vi "MainTestDemo.vi"() -> ()   [LabVIEW 2012]
uses:
  <userlib>/ROSforLV/ROS/Code/SubVIs/_ROSDirection.ctl
  <userlib>/ROSforLV/ROS/Code/_ROSDefinition.vi
  <userlib>/ROSforLV/ROS/parsing/std_msgs/subs/parse_time_scalar.vi
panel:
  in  "Tab Control":T1(tab)
  out "Time":cluster{"secs":i32, "nsecs":i32}
  in  "Load Boxes":bool
  out "WorldProperties":T2
  out "link names":string[](array[string])
  out "Link Poses":T3(array[cluster]) {"Point"."y" format="%#_3f"}
  out "Link Twists":T4(array[cluster])
  out "link names 2":string[](array[string])
  out "Link Twists 2":T4(array[cluster])
  out "Link Poses 2":T3(array[cluster]) {"Point"."y" format="%#_3f"}
  in  "Twist 2":T5
  in  "Pose 2":T6 {"Point"."x" scale=-3.0..3.0}
  in  "Pose":T6 {"Point"."x" scale=-3.0..3.0}
  in  "Twist":T5
  in  "Boolean":bool
  in  "stop":bool
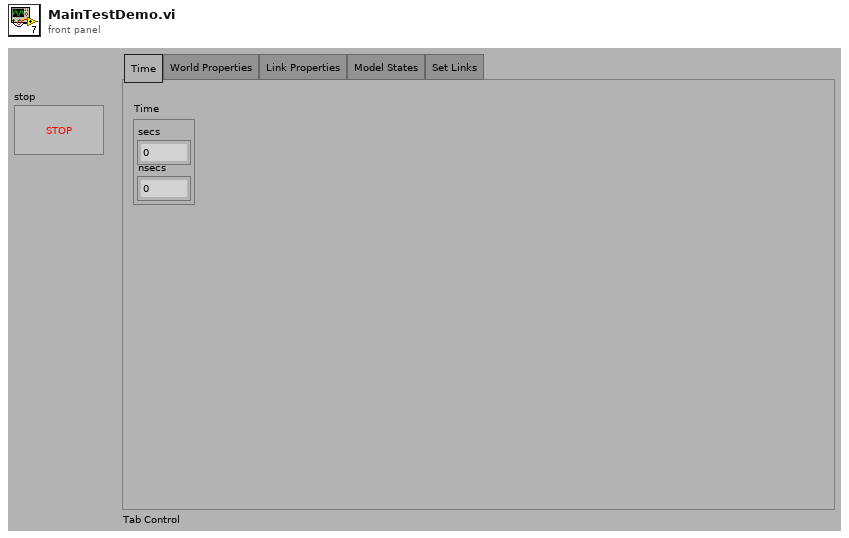
[diagram p1: front panel]
types:
  T1 = enum32{"Time", "World Properties", "Link Properties", "Model States", "Set Links"}
  T2 = cluster{"sim_time":dbl, "model_names":string[], "rendering enabled":bool, "success":bool, "status message":string}
  T3 = cluster{"Point":cluster{"x":dbl, "y":dbl, "z":dbl}, "Quaternion":cluster{"x":dbl, "y":dbl, "z":dbl, "w":dbl}}[]
  T4 = cluster{"Linear":cluster{"x":dbl, "y":dbl, "z":dbl}, "Angular":cluster{"x":dbl, "y":dbl, "z":dbl}}[]
  T5 = cluster{"Linear":cluster{"x":dbl, "y":dbl, "z":dbl}, "Angular":cluster{"x":dbl, "y":dbl, "z":dbl}}
  T6 = cluster{"Point":cluster{"x":dbl, "y":dbl, "z":dbl}, "Quaternion":cluster{"x":dbl, "y":dbl, "z":dbl, "w":dbl}}
  T7 = typedef "_ROSDirection.ctl" = enum16{"Node", "Publisher", "Subscriber", "Service Client"}
  T8 = cluster{"Topic":string, "Type":string, "Action":T7, "Update (ms)":u16, "write queue":u16}
  T9 = typedef "_ROSControl.ctl" = cluster{"topic port":u16, "Node":string, "topic":string, "type":string, "node port":u32, "error ":errorcluster, "Direction":T7, "APIs":string[], "Update (ms)":u16, "write queue":u16}
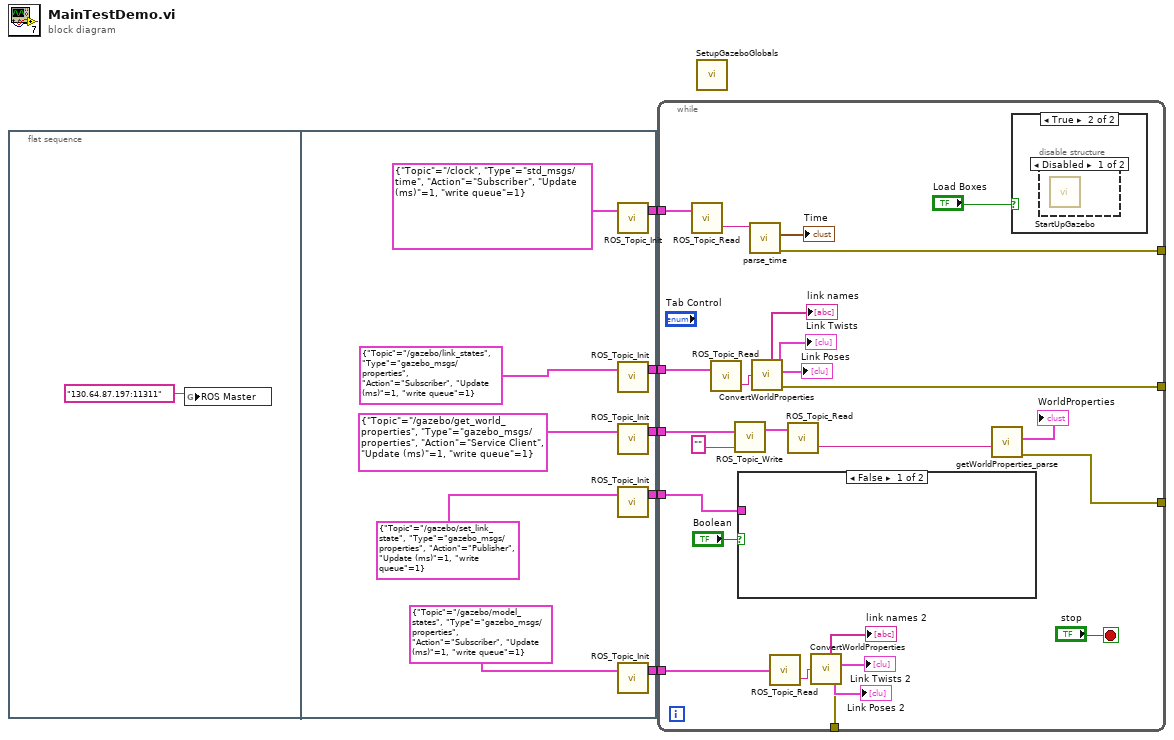
[diagram p0: block diagram]
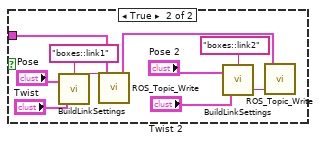
[diagram p2: hidden frame]
diagram:
  n1 = flat-sequence {
    tunnel: [w16] -> w5
    tunnel: [w15] -> w4
    tunnel: [w14] -> w3
    tunnel: [w13] -> w2
    tunnel: [w12] -> w1
    frame #0 {
      n2 = global write "_ROSDefinition.vi" "ROS Master"("130.64.87.197:11311" ("ROS Master")) -> ()
    }
    frame #1 {
      n3 = call <userlib>:"ROS_Topic_Init.vi"("Definitions"=T8 {"Topic"="/clock", "Type"="std_msgs/time", "Action"=enum."Subscriber", "Update (ms)"=1, "write queue"=1} ("element")) -> ("ROS out"=w16:T9)  [unwired: 2 in]
      n4 = call <userlib>:"ROS_Topic_Init.vi"("Definitions"=T8 {"Topic"="/gazebo/link_states", "Type"="gazebo_msgs/properties", "Action"=enum."Subscriber", "Update (ms)"=1, "write queue"=1} ("element")) -> ("ROS out"=w14:T9)  [unwired: 2 in]
      n5 = call <userlib>:"ROS_Topic_Init.vi"("Definitions"=T8 {"Topic"="/gazebo/get_world_properties", "Type"="gazebo_msgs/properties", "Action"=enum."Service Client", "Update (ms)"=1, "write queue"=1} ("element")) -> ("ROS out"=w15:T9)  [unwired: 2 in]
      n6 = call <userlib>:"ROS_Topic_Init.vi"("Definitions"=T8 {"Topic"="/gazebo/set_link_state", "Type"="gazebo_msgs/properties", "Action"=enum."Publisher", "Update (ms)"=1, "write queue"=1} ("element")) -> ("ROS out"=w13:T9)  [unwired: 2 in]
      n7 = call <userlib>:"ROS_Topic_Init.vi"("Definitions"=T8 {"Topic"="/gazebo/model_states", "Type"="gazebo_msgs/properties", "Action"=enum."Subscriber", "Update (ms)"=1, "write queue"=1} ("element")) -> ("ROS out"=w12:T9)  [unwired: 2 in]
    }
  }
  n8 = while {
    tunnel: w5 -> [w42]
    tunnel: w4 -> [w41]
    tunnel: w3 -> [w40]
    tunnel: [w33] -> _
    tunnel: [w32] -> _
    tunnel: w2 -> [w29]
    tunnel: [w28] -> _
    tunnel: w1 -> [w20]
    tunnel: [w19] -> _
    stop <- "stop" stop-if-true
    n9 = call <userlib>:"ROS_Topic_Read.vi"("ROS in"=w42) -> ("Reply"=w37:string)  [unwired: 1 in, 1 out]
    n10 = call <userlib>:"ROS_Topic_Read.vi"("ROS in"=w40) -> ("Reply"=w30:string)  [unwired: 1 in, 1 out]
    n11 = call <userlib>:"ROS_Topic_Write.vi"("Msg in"="", "ROS in"=w41) -> ("ROS out"=w39:T9)  [unwired: 2 in]
    n12 = case shown="False" "Boolean" {
      tunnel: w29 -> [_ w52]
      frame False {
      }
      frame True {
        n13 = call <userlib>:"BuildLinkSettings.vi"("Twist"="Twist", "Pose"="Pose", "link to move"="boxes::link1") -> ("msg out"=w51:string)  [unwired: 1 in]
        n14 = call <userlib>:"ROS_Topic_Write.vi"("Msg in"=w51, "ROS in"=w52) -> ("ROS out"=w44:T9)  [unwired: 2 in]
        n15 = call <userlib>:"BuildLinkSettings.vi"("Twist"="Twist 2", "Pose"="Pose 2", "link to move"="boxes::link2") -> ("msg out"=w43:string)  [unwired: 1 in]
        n16 = call <userlib>:"ROS_Topic_Write.vi"("Msg in"=w43, "ROS in"=w44) -> ()  [unwired: 2 in, 1 out]
      }
    }
    n17 = call-poly <userlib>:"parse_time.vi"("msg in"=w37) -> ("error out"=w33:errorcluster, "Time"=→"Time":cluster{"secs":i32, "nsecs":i32})  [unwired: 4 in, 1 out]
    n18 = call <userlib>:"ConvertWorldProperties.vi"("Reply"=w30) -> ("Poses"=→"Link Poses":T3, "Twists"=→"Link Twists":T4, "error out"=w28:errorcluster, "names"=→"link names":string[])  [unwired: 1 in]
    n19 = call <userlib>:"ROS_Topic_Read.vi"("ROS in"=w20) -> ("Reply"=w22:string)  [unwired: 1 in, 1 out]
    n20 = call <userlib>:"ROS_Topic_Read.vi"("ROS in"=w39) -> ("Reply"=w38:string)  [unwired: 1 in, 1 out]
    n21 = call <userlib>:"ConvertWorldProperties.vi"("Reply"=w22) -> ("Poses"=→"Link Poses 2":T3, "Twists"=→"Link Twists 2":T4, "error out"=w19:errorcluster, "names"=→"link names 2":string[])  [unwired: 1 in]
    n22 = call <userlib>:"getWorldProperties_parse.vi"("msg in"=w38) -> ("error out"=w32:errorcluster, "WorldProperties"=→"WorldProperties":T2)  [unwired: 8 in, 1 out]
    n23 = case shown="True" "Load Boxes" {
      frame False {
      }
      frame True {
        n24 = disable-structure shown="Disabled" {
          frame Disabled {
            n25 = call <userlib>:"StartUpGazebo.vi"() -> ()  [unwired: 12 in]
          }
          frame Enabled {
          }
        }
      }
    }
  }
  n26 = call <userlib>:"SetupGazeboGlobals.vi"() -> ()  [unwired: 4 in]
